vi "State_Machine.vi"(8 "error in (no error)":errorcluster caption="entrée d'erreur (pas d'erreur)", 11 "Get_Voltage en entrée":refnum<class "Read_Spectrum_Analyser.lvclass">) -> (0 "error out":errorcluster caption="sortie d'erreur", 2 "Json_String":string, 3 "Get_Voltage en sortie":refnum<class "Read_Spectrum_Analyser.lvclass">)   [LabVIEW 2020, in "Library Test.lvlib" / "Read_Spectrum_Analyser.lvclass"]
uses:
  Read_Spectrum_Analyser.lvclass
  C:/Users/ngarcin/OneDrive - Altyor/Standard TB/Class/Test/Test (Default)/Test (Default).lvclass
  Instrument/Instrument (Default)/Class Instrument (Default).lvclass
  Read_Spectrum_Analyser.lvclass/Read_Spectrum_Analyser.ctl
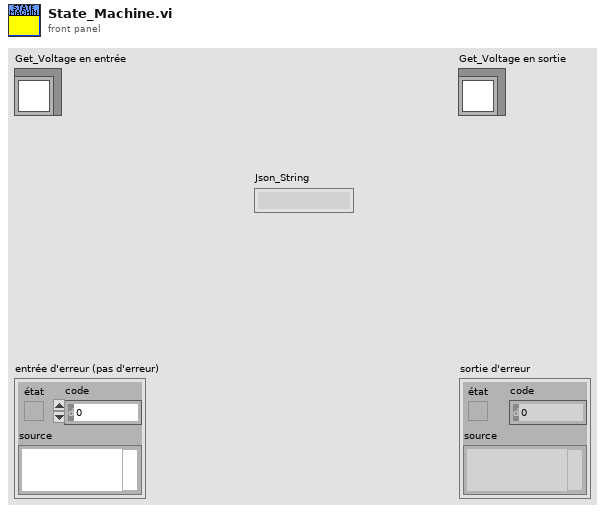
[diagram p1: front panel]
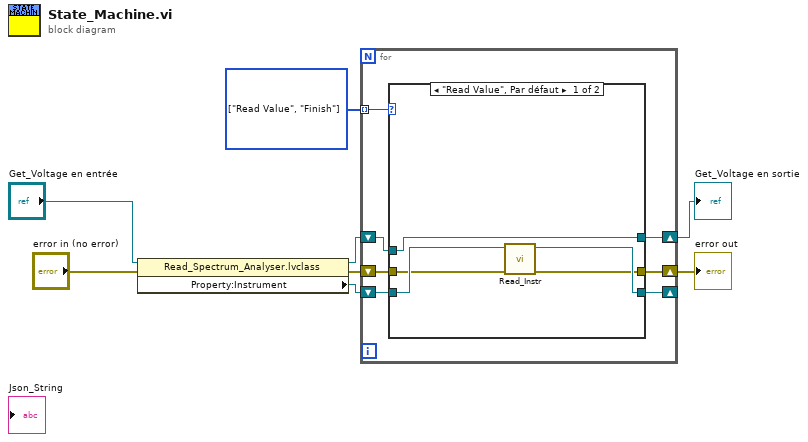
[diagram p0: block diagram]
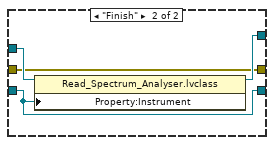
[diagram p2: hidden frame]
diagram:
  w7 = enum16{"Init", "Read Value", "Finish"}[] [enum."Read Value", enum."Finish"] items=["Init", "Read Value", "Finish"]
  n1 = property class="Read_Spectrum_Analyser.lvclass"(reference="Get_Voltage en entrée", error in="error in (no error)") -> (reference out=w5:refnum<class "Read_Spectrum_Analyser.lvclass">, error out=w1:errorcluster, "Property:Instrument"=w6:refnum<class "Class Instrument (Default).lvclass">)
  n2 = for {
    tunnel: w7 -> [w15] mode=indexing
    shift-right: [w13] -> _
    shift-left: w6 -> [w14]
    shift-right: [w11] -> w3
    shift-left: w5 -> [w12]
    shift-right: [w9] -> w4
    shift-left: w1 -> [w10]
    n3 = case shown="\"Read Value\", Par défaut" w15 {
      tunnel: w14 -> [w20 w22]
      tunnel: [w17 w22] -> w13
      tunnel: w12 -> [w18 w24]
      tunnel: [w18 w23] -> w11
      tunnel: w10 -> [w19 w21]
      tunnel: [w16 w21] -> w9
      frame "Read Value", Default {
        n4 = call-dynamic "Read_Instr.vi"("error in (no error)"=w19, "Class Instrument (Default) en entrée"=w20) -> ("error out"=w16:errorcluster, "Class Instrument (Default) en sortie"=w17:refnum<class "Class Instrument (Default).lvclass">)  [unwired: 8 in]
      }
      frame "Finish" {
        n5 = property class="Read_Spectrum_Analyser.lvclass"(reference=w24, "Property:Instrument"=w22) -> (reference out=w23:refnum<class "Read_Spectrum_Analyser.lvclass">)  [unwired: 1 in, 1 out]
      }
    }
  }
  "error out" <- w4
  "Get_Voltage en sortie" <- w3
